vi "Validate.vi"(8 "error in (no error)":errorcluster, 11 "Class in":refnum<class "Installer.lvclass">) -> (0 "error out":errorcluster, 3 "Class out":refnum<class "Installer.lvclass">)   [LabVIEW 2020, in "Installer.lvclass"]
uses:
  <vilib>/AppBuilder/IB_Classes/Installer/Installer.lvclass
  <vilib>/AppBuilder/IB_Classes/Installer/Installer.lvclass/Installer.ctl
  <resource>/Framework/Providers/Builds/Installer/CDK_GLOBAL_STRINGS.vi
  <vilib>/AppBuilder/IB_Classes/Source/IB_Source.lvclass
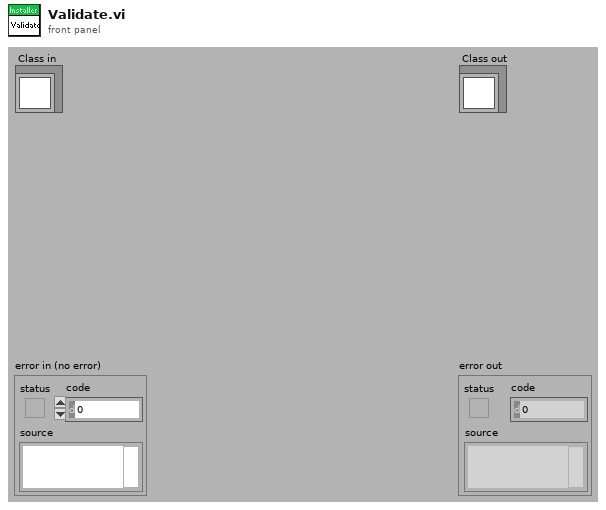
[diagram p1: front panel]
types:
  T1 = typedef "IB_Source.ctl" = cluster{"name":string, "sourceTag":string, "destTag":string, "path":path, "eng_installPath":string, "UI_inBuild?":bool, "str ref?":bool}
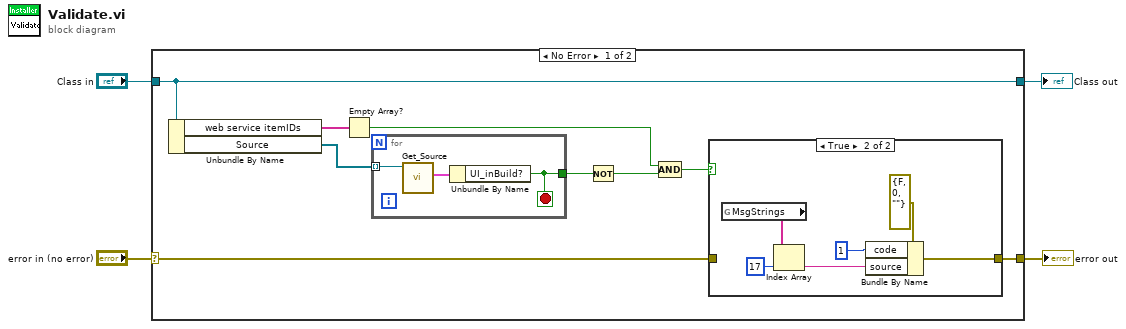
[diagram p0: block diagram]
diagram:
  n1 = case shown="No Error" "error in (no error)" {
    selector: "error in (no error)" -> [w13 w25]
    tunnel: [w12 w25] -> w3
    tunnel: [w11 w24] -> w1
    tunnel: "Class in" -> [w11 w24]
    frame No Error {
      n2 = Unbundle By Name(w11) -> ("web service itemIDs"=w8:string[], "Source"=w10:refnum<class "IB_Source.lvclass">[])
      n3 = Empty Array?(array=w8) -> (empty?=w7:bool)
      n4 = for {
        tunnel: w10 -> [w16] mode=indexing
        tunnel: [w14] -> w5
        stop <- w14 stop-if-true
        n5 = call <vilib>:"Get_Source.vi"("IB_Source in"=w16) -> ("data"=w15:T1)  [unwired: 1 in, 9 out]
        n6 = Unbundle By Name(w15) -> ("UI_inBuild?"=w14:bool)
      }
      n7 = Not(x=w5) -> (.not. x?=w6:bool)
      n8 = Compound Arithmetic op=AND(w7, w6) -> (w9:bool)
      n9 = case shown="True" w9 {
        tunnel: [w17 w19] -> w12
        tunnel: w13 -> [w17 _]
        frame False {
        }
        frame True {
          n10 = global read "CDK_GLOBAL_STRINGS.vi" "MsgStrings"() -> (w18:string[])
          n11 = Index Array(array=w18, index=17) -> (element=w20:string)
          n12 = Bundle By Name(cluster=errorcluster {"status"=FALSE, "code"=0, "source"=""} ("error IO"), "code"=1, "source"=w20) -> (w19:errorcluster)
        }
      }
    }
    frame Error {
    }
  }
  "error out" <- w3
  "Class out" <- w1
